vi "Create BitfileSpecific FpgaInterface.vi"() -> ()   [LabVIEW 2010]
panel:
  out "error out":errorcluster
  in  "New Name":string
  in  "Destination Directory":path
  in  "Bitfile Path":path
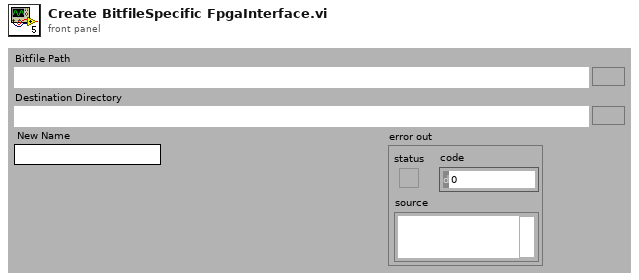
[diagram p1: front panel]
types:
  T1 = cluster{"Control Ref":refnum<vi>, "ClassID":u32, "Name":string, "VI Reference":refnum<vi>}[]
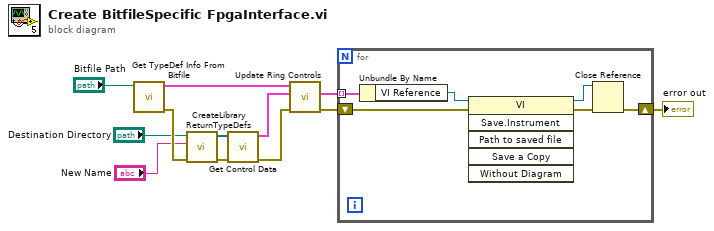
[diagram p0: block diagram]
diagram:
  n1 = call "Get TypeDef Info From Bitfile.vi"("Bitfile Path"="Bitfile Path") -> ("error out"=w9:errorcluster, "TypeDef Info"=w1:cluster{string, cluster{"Name":string, i32}[]}[])  [unwired: 9 in]
  n2 = call "CreateLibrary ReturnTypeDefs.vi"("error in (no error)"=w9, "New Name"="New Name", "Destination Directory"="Destination Directory") -> ("error out"=w5:errorcluster, "TypeDef Refs"=w4:refnum<vi>[])  [unwired: 6 in, 1 out]
  n3 = call "Get Control Data.vi"("error in (no error)"=w5, "TypeDef Refs"=w4) -> ("error out"=w2:errorcluster, "Control Data"=w3:T1)  [unwired: 8 in]
  n4 = call "Update Ring Controls.vi"("error in (no error)"=w2, "Control Data"=w3, "Parsed Header Data"=w1) -> ("error out"=w11:errorcluster, "Control Data Out"=w10:T1)  [unwired: 7 in]
  n5 = for {
    tunnel: w10 -> [w18] mode=indexing
    shift-right: [w14] -> w6
    shift-left: w11 -> [w17]
    n6 = Unbundle By Name(w18) -> ("VI Reference"=w13:refnum<vi>)
    n7 = invoke class="VI" method="Save.Instrument"(reference=w13, error in=w17) -> (reference out=w15:refnum<vi>, error out=w16:errorcluster)  [unwired: 4 in, 4 out]
    n8 = Close Reference(reference=w15, error in (no error)=w16) -> (error out=w14:errorcluster)
  }
  "error out" <- w6
